vi "Excel_Get_Names_from_Template.vi"(7 "Template File Path":path, 11 "error in (no error)":errorcluster) -> (4 "Names":string[](array[string]), 15 "error out":errorcluster)   [LabVIEW 2017, in "NI_ReportGenerationToolkit.lvlib"]
uses:
  <vilib>/addons/_office/NI_ReportGenerationToolkit.lvlib
  <vilib>/Utility/NIReport.llb/NI_ReportGenerationCore.lvlib
panel:
  in  "Excel._Application":refnum<k7>
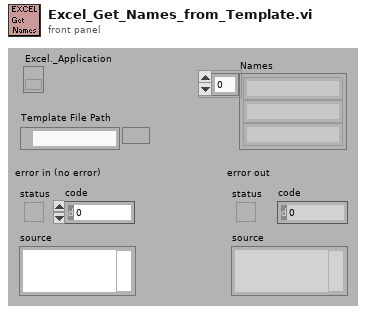
[diagram p1: front panel]
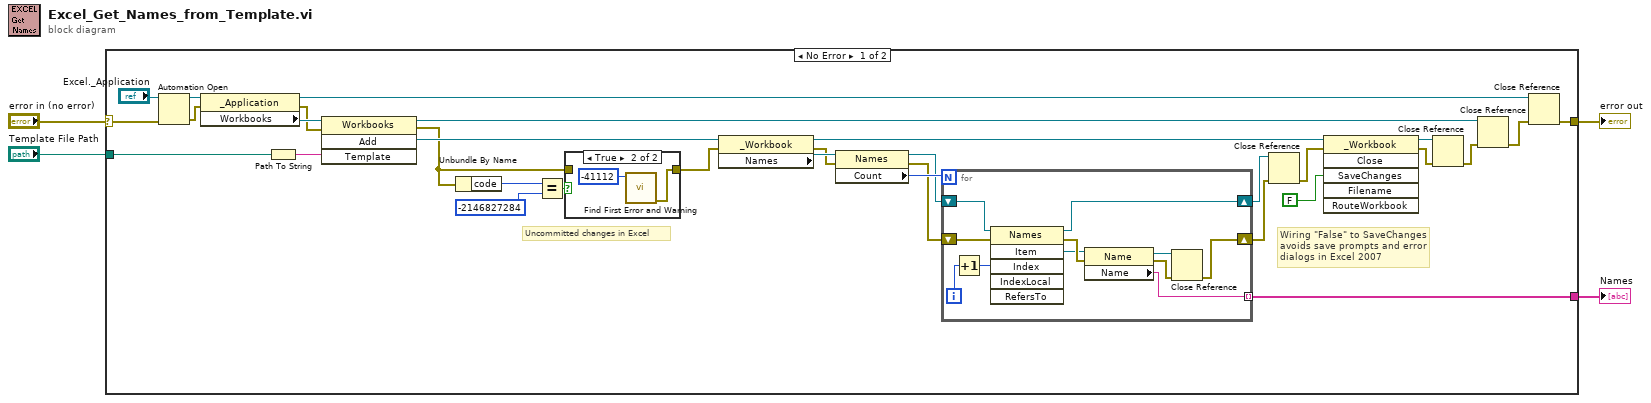
[diagram p0: block diagram]
diagram:
  n1 = case shown="No Error" "error in (no error)" {
    selector: "error in (no error)" -> [w12 w51]
    tunnel: [w36 _] -> w4
    tunnel: "Template File Path" -> [w31 _]
    tunnel: [w14 w51] -> w2
    frame No Error {
      # "Wiring \"False\" to SaveChanges\navoids save prompts and error\ndialogs in Excel 2007"
      # "Uncommitted changes in Excel"
      n2 = Automation Open(error in (no error)=w12, Automation Refnum="Excel._Application") -> (Automation Refnum=w35:refnum<k7>, error out=w34:errorcluster)  [unwired: 2 out]
      n3 = property class="_Application"(reference=w35, error in=w34) -> (reference out=w13:refnum<k7>, error out=w27:errorcluster, "Workbooks"=w28:refnum<k7>)
      n4 = Path To String(path=w31) -> (string=w30:string)
      n5 = invoke class="Workbooks" method="Add"(reference=w28, error in=w27, "Template"=w30) -> (reference out=w32:refnum<k7>, error out=w7:errorcluster, "Add"=w29:refnum<k7>)  [unwired: 1 in, 1 out]
      n6 = Unbundle By Name(w7) -> ("code"=w9:i32)
      n7 = Equal?(x=w9, y=-2146827284) -> (x = y?=w10:bool)
      n8 = case shown="True" w10 {
        tunnel: w7 -> [w37 _]
        tunnel: [w37 w39] -> w6
        frame False {
        }
        frame True {
          n9 = call <vilib>:"Find First Error and Warning.vi"("error code"=-41112 ("code")) -> ("error out"=w39:errorcluster)  [unwired: 1 in, 5 out]
        }
      }
      n10 = property class="_Workbook"(reference=w29, error in=w6) -> (reference out=w19:refnum<k7>, error out=w22:errorcluster, "Names"=w26:refnum<k7>)
      n11 = property class="Names"(reference=w26, error in=w22) -> (reference out=w23:refnum<k7>, error out=w24:errorcluster, "Count"=w25:i32)
      n12 = for {
        N: w25 -> [_]
        tunnel: [w46] -> w36 mode=indexing
        shift-right: [w43] -> w21
        shift-left: w24 -> [w45]
        shift-right: [w41] -> w20
        shift-left: w23 -> [w44]
        i -> [w49]
        n13 = Increment(x=w49) -> (x+1=w48:i32)
        n14 = invoke class="Names" method="Item"(reference=w44, error in=w45, "Index"=w48) -> (reference out=w41:refnum<k7>, error out=w50:errorcluster, "Item"=w47:refnum<k7>)  [unwired: 3 in, 3 out]
        n15 = property class="Name"(reference=w47, error in=w50) -> (reference out=w42:refnum<k7>, error out=w40:errorcluster, "Name"=w46:string)
        n16 = Close Reference(reference=w42, error in (no error)=w40) -> (error out=w43:errorcluster)
      }
      n17 = Close Reference(reference=w20, error in (no error)=w21) -> (error out=w18:errorcluster)
      n18 = invoke class="_Workbook" method="Close"(reference=w19, error in=w18, "SaveChanges"=FALSE) -> (reference out=w17:refnum<k7>, error out=w16:errorcluster)  [unwired: 3 in, 4 out]
      n19 = Close Reference(reference=w17, error in (no error)=w16) -> (error out=w33:errorcluster)
      n20 = Close Reference(reference=w32, error in (no error)=w33) -> (error out=w15:errorcluster)
      n21 = Close Reference(reference=w13, error in (no error)=w15) -> (error out=w14:errorcluster)
    }
    frame Error {
    }
  }
  "Names" <- w4
  "error out" <- w2
